vi "Stop cRIO fast measure.vi"(8 "error in (no error)":errorcluster, 10 "VI reference":refnum<vi>, 11 "application reference":refnum<vi>) -> (0 "error out":errorcluster)   [LabVIEW 2023]
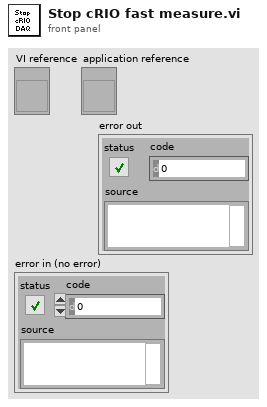
[diagram p1: front panel]
types:
  T1 = enum32{"Bad", "Idle", "Run top level", "Running"}
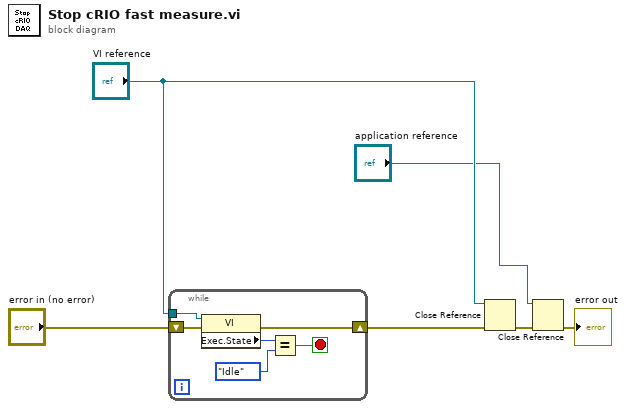
[diagram p0: block diagram]
diagram:
  n1 = while {
    tunnel: "VI reference" -> [w12]
    shift-right: [w8] -> w3
    shift-left: "error in (no error)" -> [w9]
    stop <- w7 stop-if-true
    n2 = property class="VI"(reference=w12, error in=w9) -> (error out=w8:errorcluster, "Exec.State"=w11:T1)  [unwired: 1 out]
    n3 = Equal?(x=w11, y=T1."Idle" ("Execution:State")) -> (x = y?=w7:bool)
  }
  n4 = Close Reference(reference="VI reference", error in (no error)=w3) -> (error out=w6:errorcluster)
  n5 = Close Reference(reference="application reference", error in (no error)=w6) -> (error out=→"error out":errorcluster)
